vi "TEST Multi Domain XControl.vi"() -> ()   [LabVIEW 2011]
doc: "Demonstration of an XControl.\n\nAAL 9/09"
uses:
  Multi-Graph.xctl
  <vilib>/measure/NI_MABase.lvlib
panel:
  out "Multi-Graph":waveform(dbl)(xcontrol)
  in  "Frequency":dbl(knob)=10.0 scale=0.01..500.0
  in  "stop":bool
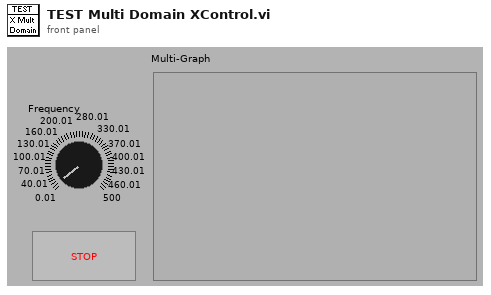
[diagram p1: front panel]
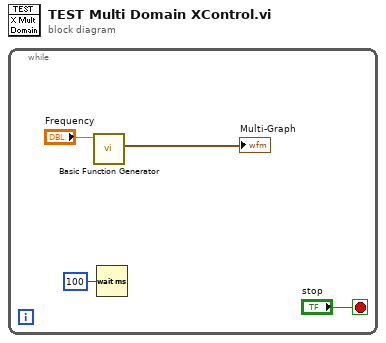
[diagram p0: block diagram]
diagram:
  n1 = while {
    stop <- "stop" stop-if-true
    n2 = call <vilib>:"Basic Function Generator.vi"("frequency"="Frequency") -> ("signal out"=→"Multi-Graph":waveform(dbl))  [unwired: 8 in, 2 out]
    n3 = Wait (ms)(milliseconds to wait=u32 100) -> ()  [unwired: 1 out]
  }
